vi "ex1-2.vi"() -> ()   [LabVIEW 2019]
panel:
  out "Waveform Chart 2":dbl(graph)
  in  "Knob 2":dbl(knob) scale=0.0..10.0
  in  "stop":bool
  in  "Knob":dbl(knob) scale=0.0..10.0
  out "Waveform Chart":dbl(graph)
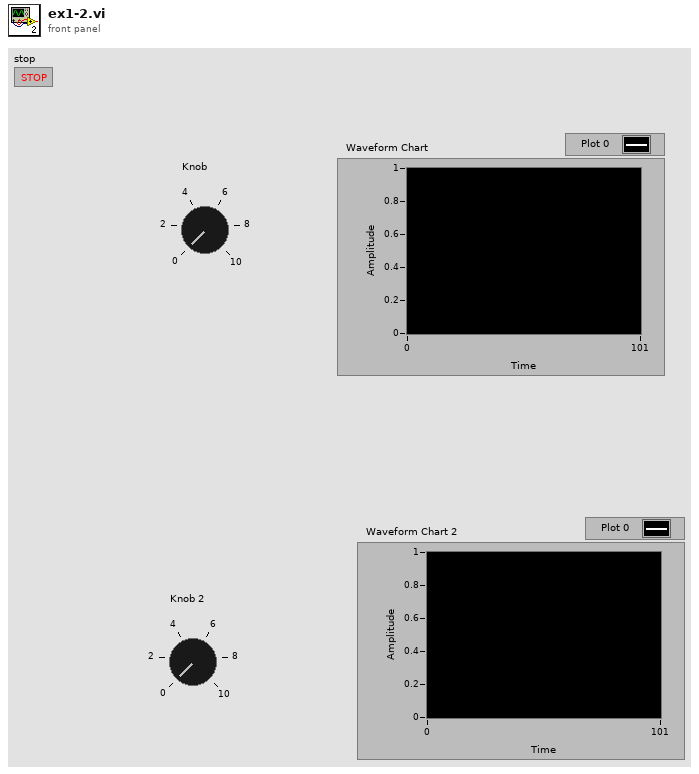
[diagram p1: front panel]
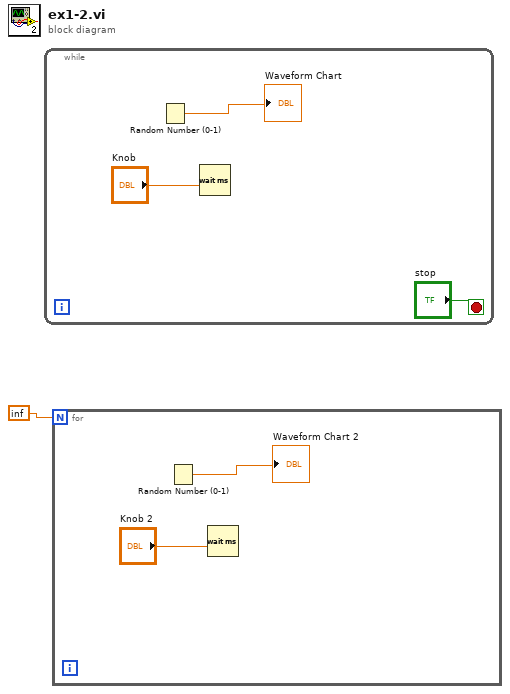
[diagram p0: block diagram]
diagram:
  n1 = while {
    stop <- "stop" stop-if-true
    n2 = Random Number (0-1)() -> (number: 0 to 1=→"Waveform Chart":dbl)
    n3 = Wait (ms)(milliseconds to wait="Knob") -> ()  [unwired: 1 out]
  }
  n4 = for {
    N: inf -> [_]
    n5 = Random Number (0-1)() -> (number: 0 to 1=→"Waveform Chart 2":dbl)
    n6 = Wait (ms)(milliseconds to wait="Knob 2") -> ()  [unwired: 1 out]
  }
